vi "Parse RS232 Data to Float.vi"(9 "AML end byte":i32, 10 "AML start byte":i32, 11 "bytes in":string) -> (2 "DBL data":dbl, 3 "bytes out":string)   [LabVIEW 2019, in "PGC2D.lvlib"]
uses:
  PGC2D.lvlib
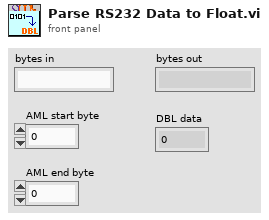
[diagram p1: front panel]
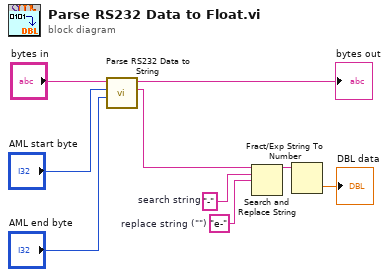
[diagram p0: block diagram]
diagram:
  w4 = "e-"  # replace string ("")
  w1 = "-"  # search string
  n1 = call "Parse RS232 Data to String.vi"("AML end byte"="AML end byte", "AML start byte"="AML start byte", "bytes in"="bytes in") -> ("string data"=w2:string, "bytes out"=→"bytes out":string)  [unwired: 7 in]
  n2 = Search and Replace String(input string=w2, search string=w1, replace string=w4) -> (result string=w5:string)  [unwired: 5 in, 3 out]
  n3 = Fract/Exp String To Number(string=w5) -> (number=→"DBL data":dbl)  [unwired: 3 in, 1 out]
